vi "bandwith.vi"() -> ()   [LabVIEW 2010]
uses:
  <vilib>/addons/PixeLINK/Low Level Functions/CAMERA_FEATURES.llb/TDPU-CameraFeatures-PixelFormat.ctl
  <vilib>/DAQmx/write.llb/DAQmx Write (Analog DBL 1Chan 1Samp).vi
  <vilib>/daqmx/miscellaneous.llb/DAQmx Fill In Error Info.vi
panel:
  out "Cuadros Tomados":i32
  in  "DAQ Parameters":T1={"Minimum Value"=-10.0, "Maximum Value"=10.0, "Physical Channel"="Dev1/ao0", "DAQ Fs (S/s)"=10000.0}
  in  "M":u32=3
  in  "N":u32=500
  in  "Tiempo estabilizacion (ms)":u32=200
  in  "Min":dbl=-10.0
  in  "Max":dbl=10.0
  out "Funciona?":bool
  in  "Analiza Señales":bool
  in  "Mete Señal":bool
  out "XY Graph":cluster{i32[], dbl[]}[](graph)
  in  "AVI Path 2":path
  in  "Tiempo":dbl
  in  "Amplitud":dbl
  in  "Freq":dbl
  in  "AVI Path":path
  in  "quality":i32=-1
  in  "AVI Compresion Filter":u16(ring) items=["Emuzed H263 Video Encoder-DMO", "Emuzed H.264 Encoder-DMO", "Emuzed MPEG-4 SP Encoder-DMO", "DV Video Encoder", "MJPEG Compressor", "Cinepak Codec by Radius", "Intel IYUV codec", "Intel IYUV codec", "Microsoft RLE", "Microsoft Video 1"]
  in  "Selector":u16(ring) items=["776002034"]
  in  "Camera Parameters":T3 {"Pixel Format" items=["PIXEL_FORMAT_MONO8", "PIXEL_FORMAT_MONO16", "PIXEL_FORMAT_YUV422", "PIXEL_FORMAT_BAYER8_GRBG", "PIXEL_FORMAT_BAYER16_GRBG", "PIXEL_FORMAT_RGB24", "PIXEL_FORMAT_RGB48", "PIXEL_FORMAT_BAYER8_RGGB", "PIXEL_FORMAT_BAYER8_GBRG ", "PIXEL_FORMAT_BAYER8_BGGR ", "PIXEL_FORMAT_BAYER16_RGGB ", "PIXEL_FORMAT_BAYER16_GBRG", "PIXEL_FORMAT_BAYER16_BGGR", "PIXEL_FORMAT_RGB32"]}
  in  "Graba Video Inicial":bool
  in  "Streeam?":bool
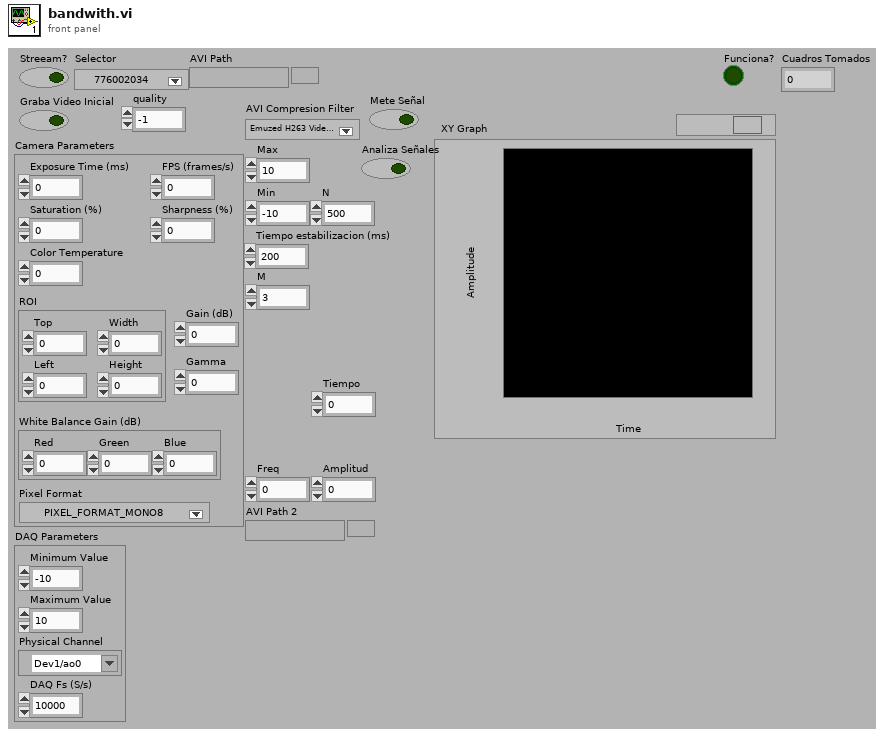
[diagram p1: front panel]
types:
  T1 = cluster{"Minimum Value":dbl, "Maximum Value":dbl, "Physical Channel":tag, "DAQ Fs (S/s)":dbl}
  T2 = typedef "TDPU-CameraFeatures-PixelFormat.ctl" = u16
  T3 = cluster{"Exposure Time (ms)":dbl, "Gain (dB)":dbl, "Saturation (%)":dbl, "Sharpness (%)":dbl, "Color Temperature":dbl, "ROI":cluster{"Top":i32, "Left":i32, "Width":i32, "Height":i32}, "White Balance Gain (dB)":cluster{"Red":dbl, "Green":dbl, "Blue":dbl}, "Gamma":dbl, "Pixel Format":T2, "FPS (frames/s)":i32}
  T4 = cluster{"hCamera":u32, "Error":errorcluster, "uSerialNumber":u32}
  T5 = cluster{"DAQ Fs (S/s)":dbl, "task":refnum<k21>, "error":errorcluster, "Min Value":dbl, "Max Value":dbl}
  T6 = typedef "AviRefnum.ctl" = refnum<k1>
  T7 = typedef "IMAQ Image.ctl" = refnum<image>
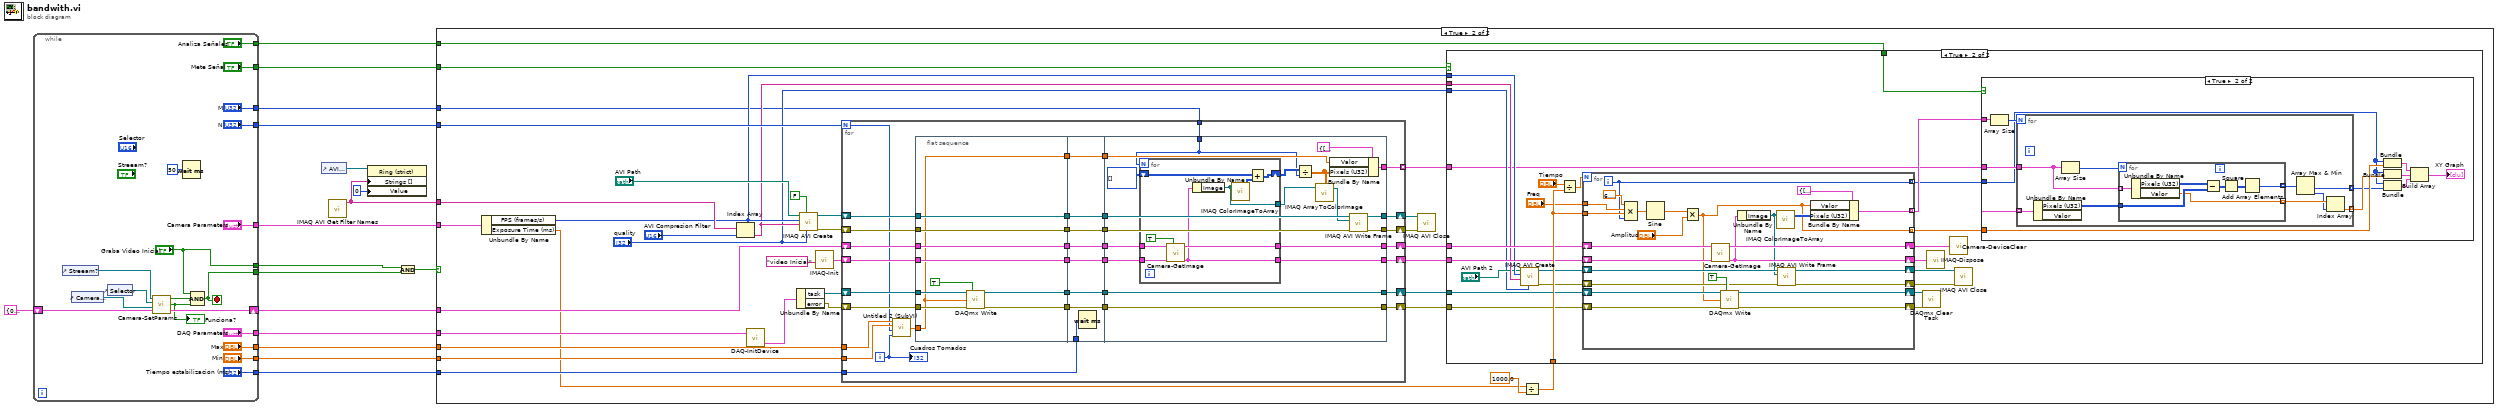
[diagram p0: block diagram]
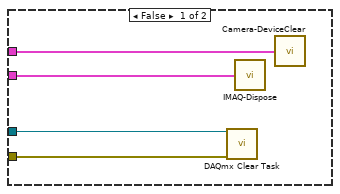
[diagram p3: hidden frame]
diagram:
  n1 = while {
    shift-right: [w36] -> w13
    shift-left: T4 {"hCamera"=0, "Error"={"status"=FALSE, "code"=0, "source"=""}, "uSerialNumber"=0} ("Camera Device OUT") -> [w35]
    tunnel: [w29] -> w11
    tunnel: ["Camera Parameters"] -> w10
    tunnel: ["Graba Video Inicial"] -> w9
    tunnel: ["N"] -> w8
    tunnel: ["DAQ Parameters"] -> w7
    tunnel: ["Max"] -> w6
    tunnel: ["Min"] -> w5
    tunnel: ["Tiempo estabilizacion (ms)"] -> w4
    tunnel: ["Mete Señal"] -> w3
    tunnel: ["Analiza Señales"] -> w2
    tunnel: ["M"] -> w1
    stop <- w29 stop-if-true
    n2 = control-ref of="Streeam?"() -> (w32:refnum<vi>)
    n3 = control-ref of="Camera Parameters"() -> (w34:refnum<vi>)
    n4 = control-ref of="Selector"() -> (w33:refnum<vi>)
    n5 = call "Camera-SetParams.vi"("Camera Device  IN"=w35, "Camera Parameters"=w34, "Selector"=w33, "Stream?"=w32) -> ("Camera Device OUT"=w36:T4, "Funciona?"=w31:bool, "Stream? OUT"=w30:bool)
    "Funciona?" <- w31
    n6 = Wait (ms)(milliseconds to wait=u32 50) -> ()  [unwired: 1 out]
    n7 = Compound Arithmetic op=AND("Graba Video Inicial", w30, w31) -> (w29:bool)
  }
  n8 = control-ref of="AVI Compresion Filter"() -> (w15:refnum<vi>)
  n9 = call "IMAQ AVI Get Filter Names"() -> ("Filter Names"=w17:string[])  [unwired: 10 in, 1 out]
  n10 = property on="Property Node" class="Ring (strict)"(reference=w15, "Strings []"=w17, "Value"=u16 0) -> ()  [unwired: 1 in, 2 out]
  n11 = And(x=w9, y=w11) -> (x .and. y?=w12:bool)
  n12 = case shown="True" w12 {
    tunnel: w5 -> [_ w70]
    tunnel: w6 -> [_ w69]
    tunnel: w4 -> [_ w68]
    tunnel: w17 -> [_ w66]
    tunnel: w8 -> [_ w56]
    tunnel: w10 -> [_ w53]
    tunnel: w7 -> [_ w52]
    tunnel: w13 -> [_ w44]
    tunnel: w3 -> [_ w42]
    tunnel: w2 -> [_ w41]
    tunnel: w1 -> [_ w40]
    frame False {
    }
    frame True {
      n13 = Unbundle By Name(w53) -> ("FPS (frames/s)"=w47:i32, "Exposure Time (ms)"=w38:dbl)
      n14 = Index Array(array=w66, index="AVI Compresion Filter") -> (element=w46:string)
      n15 = call "DAQ-InitDevice.vi"("DAQ Parameters"=w52) -> ("DAQ Device OUT"=w57:T5)  [unwired: 1 in, 2 out]
      n16 = Unbundle By Name(w57) -> ("task"=w58:refnum<k21>, "error"=w59:errorcluster)
      n17 = call "IMAQ AVI Create"("quality"="quality", "Has Data"=FALSE, "Compression Filter"=w46, "Frames Per Second"=w47, "AVI Path"="AVI Path") -> ("error out"=w61:errorcluster, "Avi Refnum"=w62:T6)  [unwired: 5 in]
      n18 = call "IMAQ-Init.vi"("Image Name"="video Inicial") -> ("Image Device IN"=w64:cluster{"Image":T7, "errorImage":errorcluster})
      n19 = for {
        N: w56 -> [w156]
        tunnel: w70 -> [w183]
        tunnel: w69 -> [w182]
        shift-right: [w160] -> w50
        shift-left: w59 -> [w180]
        shift-right: [w157] -> w51
        shift-left: w58 -> [w185]
        tunnel: w68 -> [w179]
        shift-right: [w177] -> w49
        shift-left: w44 -> [w166]
        shift-right: [w178] -> w48
        shift-left: w64 -> [w165]
        shift-right: [w176] -> w55
        shift-left: w62 -> [w169]
        shift-right: [w175] -> w54
        shift-left: w61 -> [w172]
        tunnel: w40 -> [w155]
        tunnel: [w154] -> w45 mode=indexing
        i -> [w184]
        n20 = call "Untitled 2 (SubVI).vi"("x"=w184, "N"=w156, "Min"=w183, "Max"=w182) -> ("y"=w181:dbl)
        n21 = flat-sequence {
          tunnel: w185 -> [w194]
          tunnel: w181 -> [w186]
          tunnel: w180 -> [w193]
          tunnel: [w192] -> w173
          tunnel: w172 -> [w192]
          tunnel: [w191] -> w170
          tunnel: w169 -> [w191]
          tunnel: [w190] -> w167
          tunnel: w166 -> [w190]
          tunnel: w165 -> [w189]
          tunnel: [w189] -> w163
          tunnel: [w188] -> w161
          tunnel: [w187] -> w158
          tunnel: [w186] -> w153
          tunnel: w179 -> [w203]
          tunnel: [w202] -> w174
          tunnel: w173 -> [w202]
          tunnel: [w201] -> w171
          tunnel: w170 -> [w201]
          tunnel: [w200] -> w168
          tunnel: w167 -> [w200]
          tunnel: [w199] -> w164
          tunnel: w163 -> [w199]
          tunnel: [w198] -> w162
          tunnel: w161 -> [w198]
          tunnel: [w197] -> w159
          tunnel: w158 -> [w197]
          tunnel: w153 -> [w196]
          tunnel: [w196] -> w152
          tunnel: [w221] -> w178
          tunnel: [w222] -> w177
          tunnel: [w220] -> w176
          tunnel: [w219] -> w175
          tunnel: w174 -> [w218]
          tunnel: w171 -> [w217]
          tunnel: w168 -> [w216]
          tunnel: w164 -> [w215]
          tunnel: [w214] -> w157
          tunnel: w162 -> [w214]
          tunnel: [w213] -> w160
          tunnel: w159 -> [w213]
          tunnel: w155 -> [w204]
          tunnel: [w208] -> w154
          tunnel: w152 -> [w206]
          frame #0 {
            n22 = call-poly <vilib>:"DAQmx Write.vi"("task/channels in"=w194, "auto start"=TRUE, "data"=w186, "error in"=w193) -> ("task out"=w188:refnum<k21>, "error out"=w187:errorcluster)  [unwired: 9 in, 1 out]
          }
          frame #1 {
            n23 = Wait (ms)(milliseconds to wait=w203) -> ()  [unwired: 1 out]
          }
          frame #2 {
            n24 = for {
              N: w204 -> [_]
              tunnel: [w230] -> w222
              tunnel: [w229] -> w221
              tunnel: w216 -> [w228]
              tunnel: w215 -> [w227]
              shift-right: [w225] -> w205
              shift-left: u32[][] [] -> [w224]
              tunnel: [w223] -> w211
              n25 = call "Camera-GetImage.vi"("Streeam"=TRUE, "Image Device IN"=w227, "Camera Device IN"=w228) -> ("Image Device OUT"=w229:cluster{"Image":T7, "errorImage":errorcluster}, "Camera Device OUT"=w230:T4)  [unwired: 4 in]
              n26 = Unbundle By Name(w229) -> ("Image"=w223:T7)
              n27 = call "IMAQ ColorImageToArray"("Image"=w223) -> ("Image Pixels (U32)"=w226:u32[][])  [unwired: 3 in, 2 out]
              n28 = Add(x=w224, y=w226) -> (x+y=w225:u32[][])
            }
            n29 = Divide(x=w205, y=w204) -> (x/y=w207:dbl[][])
            n30 = call "IMAQ ArrayToColorImage"("Image Pixels (U32)"=w207, "Image"=w211) -> ("Image Out"=w210:T7)  [unwired: 3 in, 1 out]
            n31 = Bundle By Name(cluster=cluster{"Pixels (U32)":u32[][], "Valor":dbl} {"Pixels (U32)"=[], "Valor"=0.0} ("input cluster"), "Valor"=w206, "Pixels (U32)"=w207) -> (w208:cluster{"Pixels (U32)":u32[][], "Valor":dbl})
            n32 = call "IMAQ AVI Write Frame"("error in (no error)"=w218, "Image"=w210, "Avi Refnum"=w217) -> ("error out"=w219:errorcluster, "Avi Refnum (duplicate)"=w220:T6)  [unwired: 7 in]
          }
        }
        "Cuadros Tomados" <- w184
      }
      n33 = call "IMAQ AVI Close"("error in (no error)"=w54, "Avi Refnum"=w55) -> ()  [unwired: 9 in, 1 out]
      n34 = Divide(x=w38, y=1000.0) -> (x/y=w37:dbl)
      n35 = case shown="True" w42 {
        tunnel: w37 -> [_ w97]
        tunnel: w51 -> [w72 w96]
        tunnel: w50 -> [w71 w95]
        tunnel: w49 -> [w74 w93]
        tunnel: w48 -> [w73 w92]
        tunnel: w47 -> [_ w89]
        tunnel: w46 -> [_ w88]
        tunnel: "quality" -> [_ w86]
        tunnel: w45 -> [_ w78]
        tunnel: w41 -> [_ w75]
        frame False {
          n36 = call <vilib>:"DAQmx Clear Task.vi"("task in"=w72, "error in"=w71) -> ()  [unwired: 13 in, 1 out]
          n37 = call "IMAQ-Dispose.vi"("Image Device IN"=w73) -> ()
          n38 = call "Camera-DeviceClear.vi"("Camera Device OUT"=w74) -> ()
        }
        frame True {
          n39 = call "IMAQ AVI Create"("quality"=w86, "Compression Filter"=w88, "Frames Per Second"=w89, "AVI Path"="AVI Path 2") -> ("error out"=w90:errorcluster, "Avi Refnum"=w91:T6)  [unwired: 6 in]
          n40 = Divide(x="Tiempo", y=w97) -> (x/y=w99:dbl)
          n41 = for {
            N: w99 -> [_]
            tunnel: w97 -> [w147]
            tunnel: "Freq" -> [w143]
            shift-right: [w142] -> w81
            shift-left: w96 -> [w145]
            shift-right: [w141] -> w80
            shift-left: w95 -> [w144]
            shift-right: [w138] -> w83
            shift-left: w93 -> [w140]
            shift-right: [w137] -> w82
            shift-left: w92 -> [w139]
            shift-right: [w133] -> w85
            shift-left: w91 -> [w136]
            shift-right: [w132] -> w84
            shift-left: w90 -> [w135]
            tunnel: [w130] -> w79 mode=indexing
            tunnel: [w128] -> w77 mode=indexing
            tunnel: [w127] -> w76 mode=indexing
            i -> [w127]
            n42 = Compound Arithmetic op=MULTIPLY(6.283185307179586, w143, w147, w127) -> (w149:dbl)
            n43 = Sine(x=w149) -> (sin(x)=w150:dbl)
            n44 = Multiply(x=w150, y="Amplitud") -> (x*y=w128:dbl)
            n45 = call "Camera-GetImage.vi"("Image Device IN"=w139, "Camera Device IN"=w140) -> ("Image Device OUT"=w137:cluster{"Image":T7, "errorImage":errorcluster}, "Camera Device OUT"=w138:T4)  [unwired: 5 in]
            n46 = call-poly <vilib>:"DAQmx Write.vi"("task/channels in"=w145, "auto start"=TRUE, "data"=w128, "error in"=w144) -> ("task out"=w142:refnum<k21>, "error out"=w141:errorcluster)  [unwired: 9 in, 1 out]
            n47 = Unbundle By Name(w137) -> ("Image"=w134:T7)
            n48 = call "IMAQ ColorImageToArray"("Image"=w134) -> ("Image Pixels (U32)"=w131:u32[][])  [unwired: 3 in, 2 out]
            n49 = call "IMAQ AVI Write Frame"("error in (no error)"=w135, "Image"=w134, "Avi Refnum"=w136) -> ("error out"=w132:errorcluster, "Avi Refnum (duplicate)"=w133:T6)  [unwired: 7 in]
            n50 = Bundle By Name(cluster=cluster{"Pixels (U32)":u32[][], "Valor":dbl} {"Pixels (U32)"=[], "Valor"=0.0} ("input cluster"), "Valor"=w128, "Pixels (U32)"=w131) -> (w130:cluster{"Pixels (U32)":u32[][], "Valor":dbl})
          }
          n51 = call <vilib>:"DAQmx Clear Task.vi"("task in"=w81, "error in"=w80) -> ()  [unwired: 13 in, 1 out]
          n52 = call "IMAQ-Dispose.vi"("Image Device IN"=w82) -> ()
          n53 = call "Camera-DeviceClear.vi"("Camera Device OUT"=w83) -> ()
          n54 = call "IMAQ AVI Close"("error in (no error)"=w84, "Avi Refnum"=w85) -> ()  [unwired: 9 in, 1 out]
          n55 = case shown="True" w75 {
            tunnel: w79 -> [_ w109]
            tunnel: w78 -> [_ w108]
            tunnel: w77 -> [_ w104]
            tunnel: w76 -> [_ w101]
            frame False {
            }
            frame True {
              n56 = Array Size(array=w109) -> (size(s)=w110:i32)
              n57 = for {
                N: w110 -> [_]
                tunnel: w109 -> [w119] mode=indexing
                tunnel: w108 -> [w117]
                tunnel: [w112] -> w100 mode=indexing
                tunnel: [w111] -> w103 mode=indexing
                n58 = Unbundle By Name(w119) -> ("Pixels (U32)"=w116:u32[][])  [unwired: 1 out]
                n59 = Array Size(array=w117) -> (size(s)=w118:i32)
                n60 = for {
                  N: w118 -> [_]
                  tunnel: w117 -> [w126] mode=indexing
                  tunnel: w116 -> [w124]
                  tunnel: [w121] -> w115 mode=indexing
                  tunnel: [w120] -> w114 mode=indexing
                  n61 = Unbundle By Name(w126) -> ("Pixels (U32)"=w125:u32[][], "Valor"=w120:dbl)
                  n62 = Subtract(x=w125, y=w124) -> (x-y=w123:u32[][])
                  n63 = Square(x=w123) -> (x^2=w122:u32[][])
                  n64 = Add Array Elements(numeric array=w122) -> (sum=w121:u32)
                }
                n65 = Array Max & Min(array=w115) -> (min value=w112:u32, min index (indices)=w113:i32)  [unwired: 2 out]
                n66 = Index Array(array=w114, index=w113) -> (element=w111:dbl)
              }
              n67 = Bundle(w101, w104) -> (w106:cluster{i32[], dbl[]})  [unwired: 1 in]
              n68 = Bundle(w101, w103) -> (w107:cluster{i32[], dbl[]})  [unwired: 1 in]
              n69 = Bundle(w101, w100) -> (w102:cluster{i32[], u32[]})  [unwired: 1 in]
              n70 = Build Array(w106, w107, w102) -> (→"XY Graph":cluster{i32[], dbl[]}[])
            }
          }
        }
      }
    }
  }
